vi "camera_do_waveform_multiD.vi"(0 "Actual Sweep Time (µS)":u32, 5 "Sweep Interval (µS)":u32, 7 "Number of Slices":u32, 9 "Left Padding":u32, 11 "Right Padding":u32, 12 "Resolution":dbl) -> (8 "Digital Waveform Graph":digitalwaveform(graph))   [LabVIEW 2013]
uses:
  <vilib>/Waveform/DWDTOps.llb/Digital Pattern Generator (Single Value).vi
  <vilib>/Waveform/DWDTOps.llb/DWDT Append Digital Samples.vi
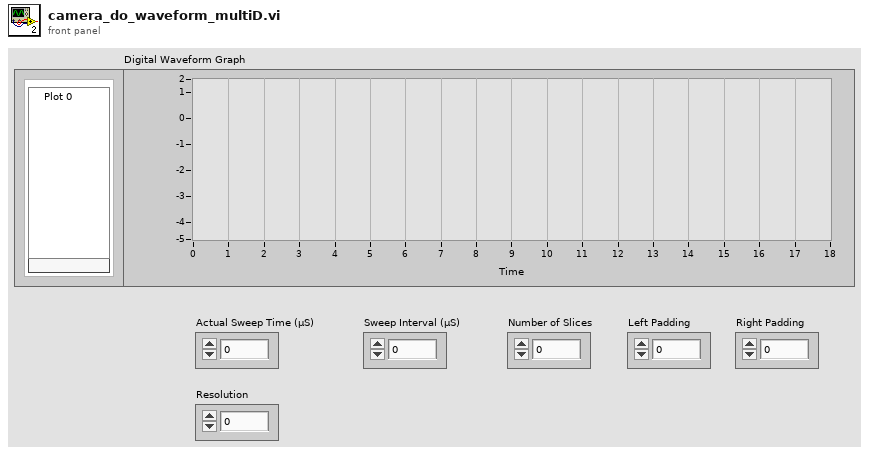
[diagram p1: front panel]
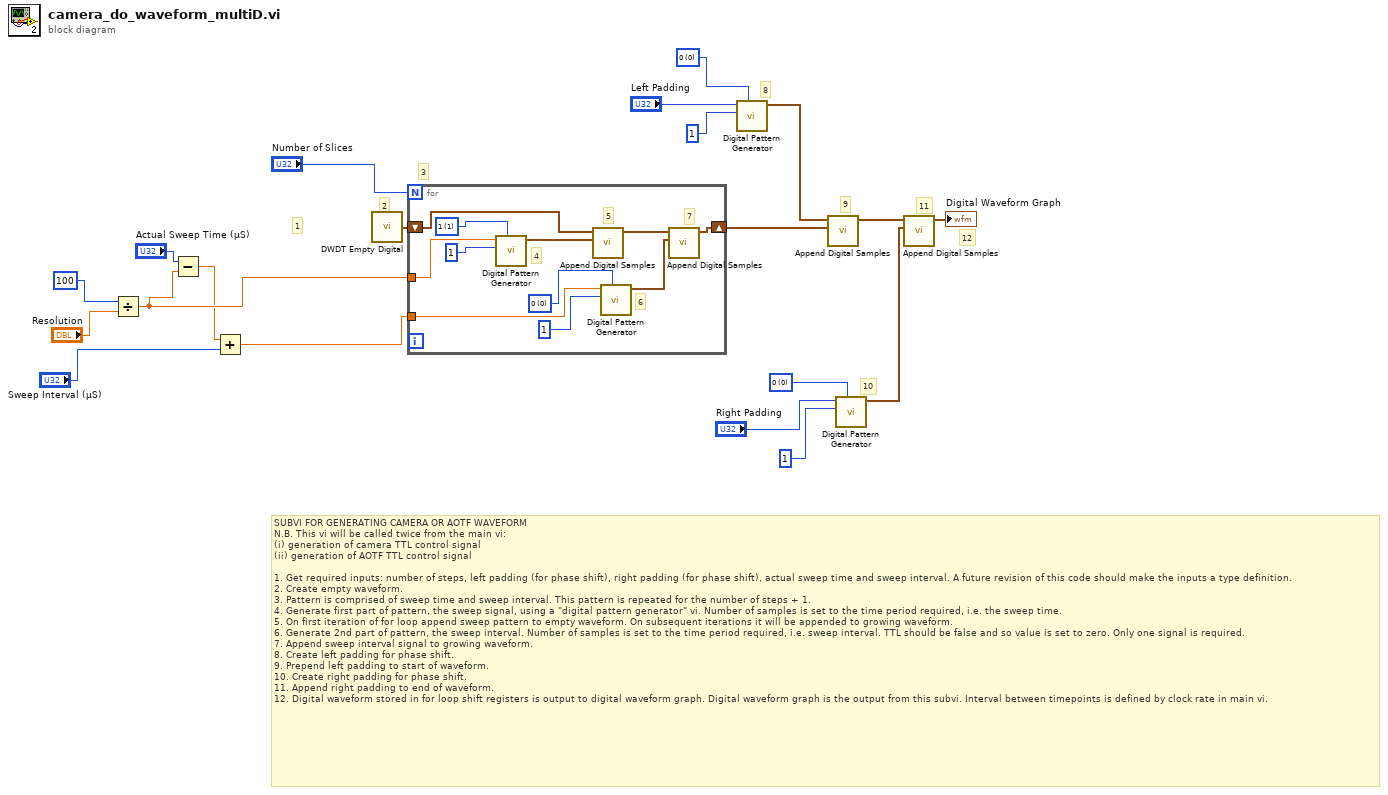
[diagram p0: block diagram]
diagram:
  w14 = u8 0 items=["0", "1", "Z", "L", "H", "X", "T", "V"] ("value")
  w17 = u8 0 items=["0", "1", "Z", "L", "H", "X", "T", "V"] ("value")
  # "12"
  # "11"
  # "10"
  # "9"
  # "8"
  # "3"
  # "2"
  # "1"
  # "SUBVI FOR GENERATING CAMERA OR AOTF WAVEFORM\nN.B. This vi will be called twice from the main vi: \n(i) generation of camera TTL control signal\n(ii) generation of AOTF TTL control signal\n\n1. Get required inputs: number of steps, left padding (for phase shift), right padding (for phase shift), actual sweep time and sweep interval. A future revision of this code should make the inputs a type definition.\n2. Create empty waveform.\n3. Pattern is comprised of sweep time and sweep interval. This pattern is repeated for the number of steps + 1.\n4. Generate first part of pattern, the sweep signal, using a \"digital pattern generator\" vi. Number of samples is set to the time period required, i.e. the sweep time.\n5. On first iteration of for loop append sweep pattern to empty waveform. On subsequent iterations it will be appended to growing waveform.\n6. Generate 2nd part of pattern, the sweep interval. Number of samples is set to the time period required, i.e. sweep interval. TTL should be false and so value is set to zero. Only one signal is required. \n7. Append sweep interval signal to growing waveform.\n8. Create left padding for phase shift.\n9. Prepend left padding to start of waveform.\n10. Create right padding for phase shift.\n11. Append right padding to end of waveform.\n12. Digital waveform stored in for loop shift registers is output to digital waveform graph. Digital waveform graph is the output from this subvi. Interval between timepoints is defined by clock rate in main vi."
  n1 = Divide(x=100, y="Resolution") -> (x/y=w4:dbl)
  n2 = Subtract(x="Actual Sweep Time (µS)", y=w4) -> (x-y=w2:dbl)
  n3 = Add(x=w2, y="Sweep Interval (µS)") -> (x+y=w1:dbl)
  n4 = call <vilib>:"DWDT Empty Digital.vi"() -> ("digital waveform out"=w20:digitalwaveform)  [unwired: 5 in]
  n5 = for {
    N: "Number of Slices" -> [_]
    shift-right: [w21] -> w12
    shift-left: w20 -> [w22]
    tunnel: w4 -> [w25]
    tunnel: w1 -> [w24]
    w29 = u8 0 items=["0", "1", "Z", "L", "H", "X", "T", "V"] ("value")
    w31 = u8 1 items=["0", "1", "Z", "L", "H", "X", "T", "V"] ("value")
    # "7"
    # "6"
    # "5"
    # "4"
    n6 = call-poly <vilib>:"Digital Pattern Generator.vi"("value"=w31, "number of signals"=u32 1, "number of samples"=w25) -> ("digital waveform"=w27:digitalwaveform)  [unwired: 7 in, 1 out]
    n7 = call-poly <vilib>:"Append Digital Samples.vi"("digital waveform B"=w27, "digital waveform A"=w22) -> ("digital waveform out"=w26:digitalwaveform)  [unwired: 8 in, 1 out]
    n8 = call-poly <vilib>:"Digital Pattern Generator.vi"("value"=w29, "number of signals"=u32 1, "number of samples"=w24) -> ("digital waveform"=w23:digitalwaveform)  [unwired: 7 in, 1 out]
    n9 = call-poly <vilib>:"Append Digital Samples.vi"("digital waveform B"=w23, "digital waveform A"=w26) -> ("digital waveform out"=w21:digitalwaveform)  [unwired: 8 in, 1 out]
  }
  n10 = call-poly <vilib>:"Digital Pattern Generator.vi"("value"=w14, "number of signals"=u32 1, "number of samples"="Left Padding") -> ("digital waveform"=w13:digitalwaveform)  [unwired: 7 in, 1 out]
  n11 = call-poly <vilib>:"Append Digital Samples.vi"("digital waveform B"=w12, "digital waveform A"=w13) -> ("digital waveform out"=w11:digitalwaveform)  [unwired: 8 in, 1 out]
  n12 = call-poly <vilib>:"Digital Pattern Generator.vi"("value"=w17, "number of signals"=u32 1, "number of samples"="Right Padding") -> ("digital waveform"=w10:digitalwaveform)  [unwired: 7 in, 1 out]
  n13 = call-poly <vilib>:"Append Digital Samples.vi"("digital waveform B"=w10, "digital waveform A"=w11) -> ("digital waveform out"=→"Digital Waveform Graph":digitalwaveform)  [unwired: 8 in, 1 out]
